vi "DeviceNet Read Data.vi"() -> ()   [LabVIEW 2016]
uses:
  <vilib>/DeviceNet/VIAPI/subVIs/DnetIOConfig.ctl
  <vilib>/DeviceNet/DeviceNetLIB.lvlib
panel:
  in  "DeviceNet IO configuration":T1={"device MAC ID"=63, "connection type"=enum."Poll", "input length"=1, "output length"=1, "expected packet rate"=200} {"expected packet rate" step=1; "output length" max=256 step=1; "input length" max=256 step=1; "device MAC ID" max=63 step=1}
  in  "interface name":T2(ring)
  out "Error out":errorcluster={"status"=TRUE, "code"=-1074388986, "source"="Open DeviceNet Interface.vi"} {"code" format="%.0x"}
  in  "Error in":errorcluster {"code" format="%.0x"}
  in  "ByteOffset":u16
  out "String Out":string
  out "DBL/SGL Out":dbl format="%.2f"
  out "8[TF] Out":bool[](array[boolean])
  out "I32/I16/I8 Out":i32
  out "U32/U16/U8 Out":u32
  in  "Dnet Input Type":T3(ring)
  out "DnetData in":u8[](array[numeric])
  # "DeviceNet Read Data"
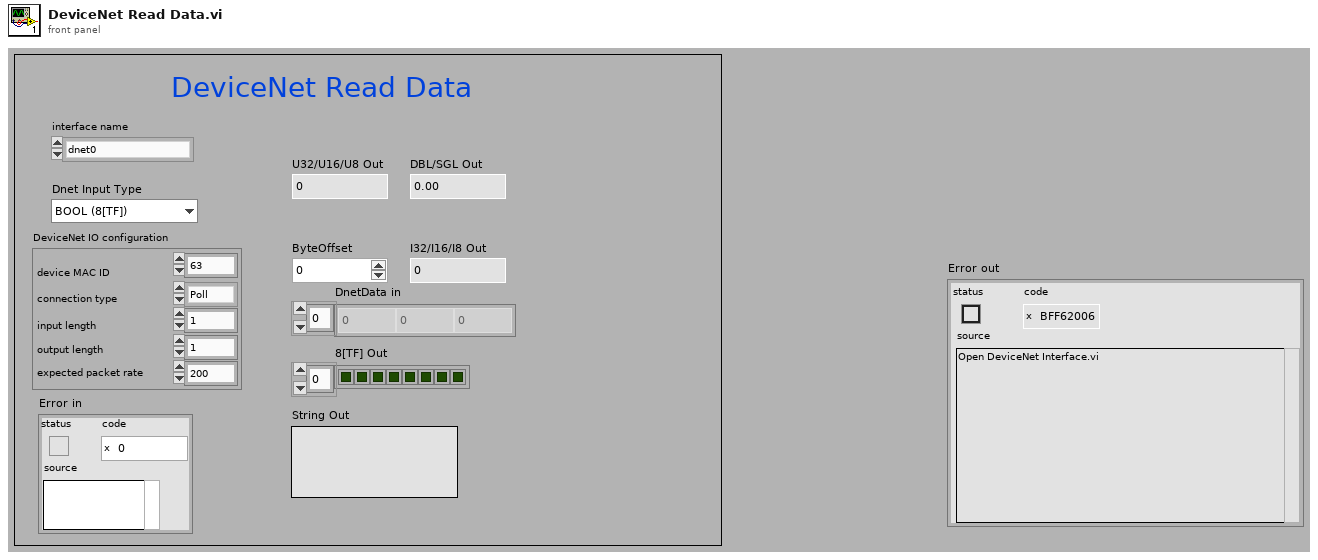
[diagram p1: front panel]
types:
  T1 = typedef "DeviceNetLIB.lvlib/DnetIOConfig.ctl" = cluster{"device MAC ID":u32, "connection type":enum32{"Poll", "Strobe", "COS", "Cyclic"}, "input length":u32, "output length":u32, "expected packet rate":u32}
  T2 = enum16{"dnet0", "dnet1", "dnet2", "dnet3", "dnet4", "dnet5", "dnet6", "dnet7", "dnet8", "dnet9", "dnet10", "dnet11", "dnet12", "dnet13", "dnet14", "dnet15", "dnet16", "dnet17", "dnet18", "dnet19", "dnet20", "dnet21", "dnet22", "dnet23", "dnet24", "dnet25", "dnet26", "dnet27", "dnet28", "dnet29", "dnet30", "dnet31"}
  T3 = enum16{"BOOL (8[TF])", "SINT (I8)", "INT (I16)", "DINT (I32)", "USINT (U8)", "UINT (U16)", "UDINT (U32)", "REAL (SGL)", "LREAL (DBL)", "SHORT_STRING (abc)", "STRING (abc)"}
  T4 = typedef "DeviceNetLIB.lvlib/xobjhandle.ctl" = u32
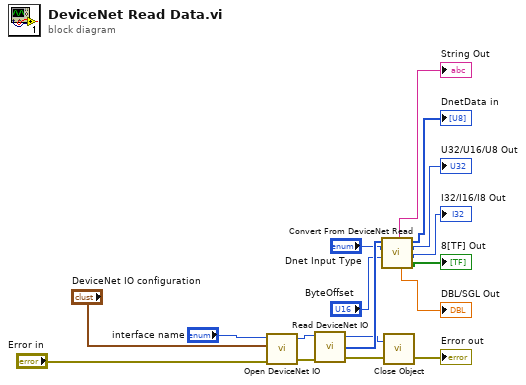
[diagram p0: block diagram]
diagram:
  n1 = call <vilib>:"Open DeviceNet IO.vi"("interface name"="interface name", "DeviceNet IO configuration"="DeviceNet IO configuration", "error in (no error)"="Error in") -> ("object handle out"=w2:T4, "error out"=w1:errorcluster)  [unwired: 4 in]
  n2 = call <vilib>:"Read DeviceNet IO.vi"("object handle in"=w2, "error in (no error)"=w1) -> ("object handle out"=w6:T4, "data"=w11:u8[], "error out"=w7:errorcluster)  [unwired: 3 in]
  n3 = call <vilib>:"Convert From DeviceNet Read.vi"("byte offset (0)"="ByteOffset", "DeviceNet type (BOOL)"="Dnet Input Type", "DeviceNet data in (0)"=w11) -> ("8 [TF] out"=→"8[TF] Out":bool[], "I32/I16/I8 out"=→"I32/I16/I8 Out":i32, "U32/U16/U8 out"=→"U32/U16/U8 Out":u32, "DeviceNet data out"=→"DnetData in":u8[], "DBL/SGL out"=→"DBL/SGL Out":dbl, "string out"=→"String Out":string)  [unwired: 3 in]
  n4 = call <vilib>:"Close Object.vi"("error in (no error)"=w7, "object handle in"=w6) -> ("error out"=→"Error out":errorcluster)  [unwired: 1 in]
